vi "Send Voltage.vi"(8 "error in":errorcluster, 11 "89XX in":refnum<class "89XX.lvclass">) -> (0 "error out":errorcluster, 3 "89XX out":refnum<class "89XX.lvclass">)   [LabVIEW 2019, in "89XX.lvlib" / "89XX.lvclass"]
uses:
  Library/89XX.lvclass
  C:/Users/Public/Documents/Development/builds/Instruments/PowerSupply.lvlibp/Library/PowerSupply.lvclass
  Library/89XX.lvclass/89XX.ctl
  Accessors/Read Local Resource.vi
  <instrlib>/Keysight N8900 Series/Keysight N8900 Series.lvlib
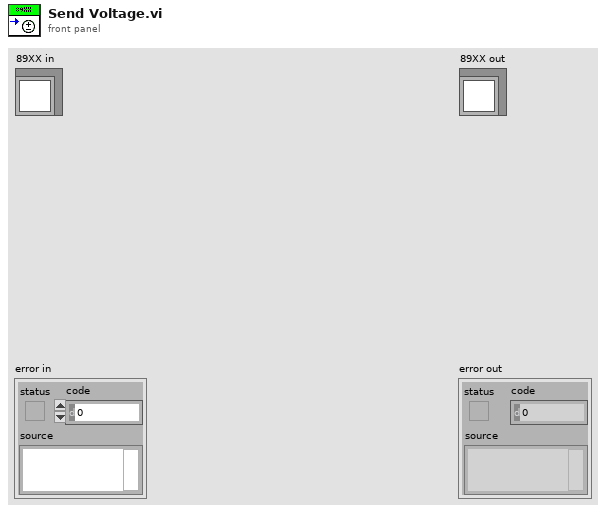
[diagram p1: front panel]
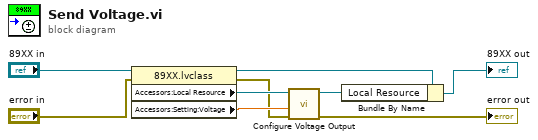
[diagram p0: block diagram]
diagram:
  n1 = property class="89XX.lvclass"(reference="89XX in", error in="error in") -> (reference out=w4:refnum<class "89XX.lvclass">, error out=w5:errorcluster, "Accessors:Local Resource"=w7:refnum<visa-resource-name>, "Accessors:Setting:Voltage"=w6:dbl)
  n2 = call <instrlib>:"Configure Voltage Output.vi"("error in (no error)"=w5, "Immediate Voltage (0 V)"=w6, "VISA resource name"=w7) -> ("error out"=→"error out":errorcluster, "VISA resource name out"=w2:refnum<visa-resource-name>)  [unwired: 7 in]
  n3 = Bundle By Name(cluster=w4, "Local Resource"=w2) -> (→"89XX out":refnum<class "89XX.lvclass">)
